vi "Config Correct CHG CLG (OptE).vi"(0 "VISA resource name":refnum<visa-resource-name>, 5 "Type (DCXTPG1)":i32(ring) items=["DCXTPG1", "TTA1"], 7 "CHG (100pF)":dbl=100.0 min=0.0 max=10000.0 step=1.0, 9 "CLG (100pF)":dbl=100.0 min=0.0 max=10000.0 step=1.0, 11 "error in":errorcluster) -> (4 "VISA resource name out":refnum<visa-resource-name>, 15 "error out":errorcluster)   [LabVIEW 2019, in "Andeen-Hagerling 2700(400 firmware).lvlib"]
doc: "Compensates for the stray HIGH-to-ground and LOW-toground capacitance of the device under test (DUT) for the DCXTPG1 and TTA1 correction types respectively.\n\nThis command is only supported on the Option-E version of the AH2700A."
uses:
  Andeen-Hagerling 2700(400 firmware).lvlib
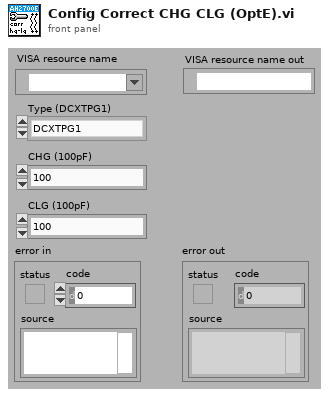
[diagram p1: front panel]
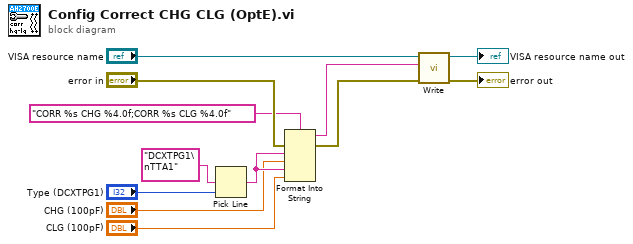
[diagram p0: block diagram]
diagram:
  n1 = Pick Line(multi-line string="DCXTPG1\nTTA1", line index="Type (DCXTPG1)") -> (output string=w3:string)  [unwired: 1 in]
  n2 = Format Into String(format string="CORR %s CHG %4.0f;CORR %s CLG %4.0f", error in="error in", w3, "CHG (100pF)", w3, "CLG (100pF)") -> (resulting string=w6:string, error out=w8:errorcluster)  [unwired: 1 in]
  n3 = call "Write.vi"("error in"=w8, "command"=w6, "VISA resource name"="VISA resource name") -> ("error out"=→"error out":errorcluster, "VISA resource name out"=→"VISA resource name out":refnum<visa-resource-name>)  [unwired: 7 in]
